vi "Servo Tracking State Machine.vi"(0 "Servo Positions In":cluster{"X":dbl, "Y":dbl}, 1 "Image Size":T4=enum."320x240", 7 "Rectangle":T3, 9 "Particles":i32, 11 "Area":i32=4) -> (4 "Servo Positions":cluster{"X":dbl, "Y":dbl}, 6 "Tracking State Info":T2)   [LabVIEW 2013]
uses:
  <vilib>/Rock Robotics/WPI/Camera/WPI_CameraImageSize.ctl
  Control States.ctl
panel:
  in  "Upper Limit":cluster{"X":i32, "Y":i32}={"X"=169, "Y"=130}
  in  "Lower Limit":cluster{"X":i32, "Y":i32}={"X"=0, "Y"=40}
  in  "Search Speed":i32=4
  in  "Proportional (div)":cluster{"X":i32, "Y":i32}={"X"=15, "Y"=-13}
  # "Unwired tuning params for control.\nSearch speed determines how fast the\ngimbal will move when trying to acquire\na target. Too fast and you may miss the\ntarget between frames, too slow is boring.\n\nProportional(div) is the proportional constant\nexpressed as a divisor term. Adjust this higher\nif the gimbal is oscillating, lower for quicker\nresponse.\n\nThe limits are useful for keeping the gimbal in\na working range, some stick when the get near\ntheir mechanical limits. It is also useful to limit\nthe searching to avoid looking at the ceiling, etc."
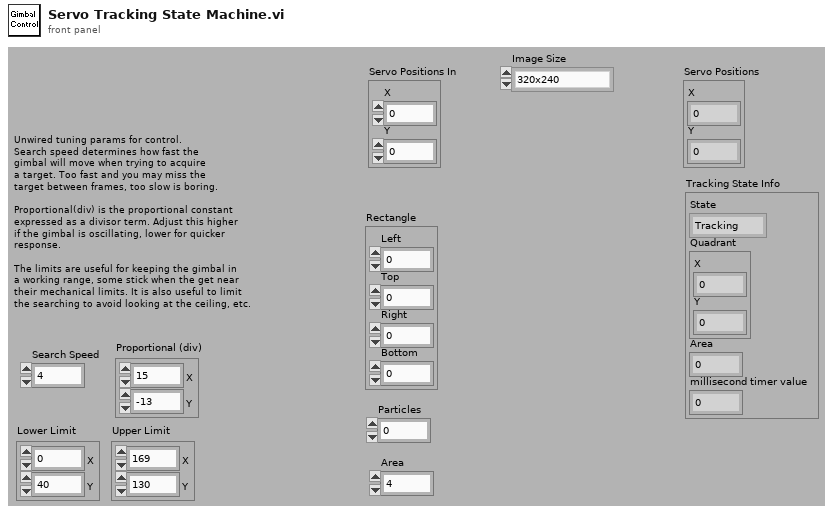
[diagram p1: front panel]
types:
  T1 = typedef "Control States.ctl" = enum16{"Tracking", "Lost Small", "Lost-Patience", "Search-Begin", "Searching", "Lost - Edge"}
  T2 = cluster{"State":T1, "Quadrant":cluster{"X":i32, "Y":i32}, "Area":i32, "millisecond timer value":u32}
  T3 = cluster{"Left":i32, "Top":i32, "Right":i32, "Bottom":i32}
  T4 = typedef "WPI_CameraImageSize.ctl" = enum16{"640x480", "320x240", "160x120"}
  T5 = cluster{"State":T1, "Grid Element":cluster{"X":i32, "Y":i32}, "Area":i32, "millisecond timer value":u32}
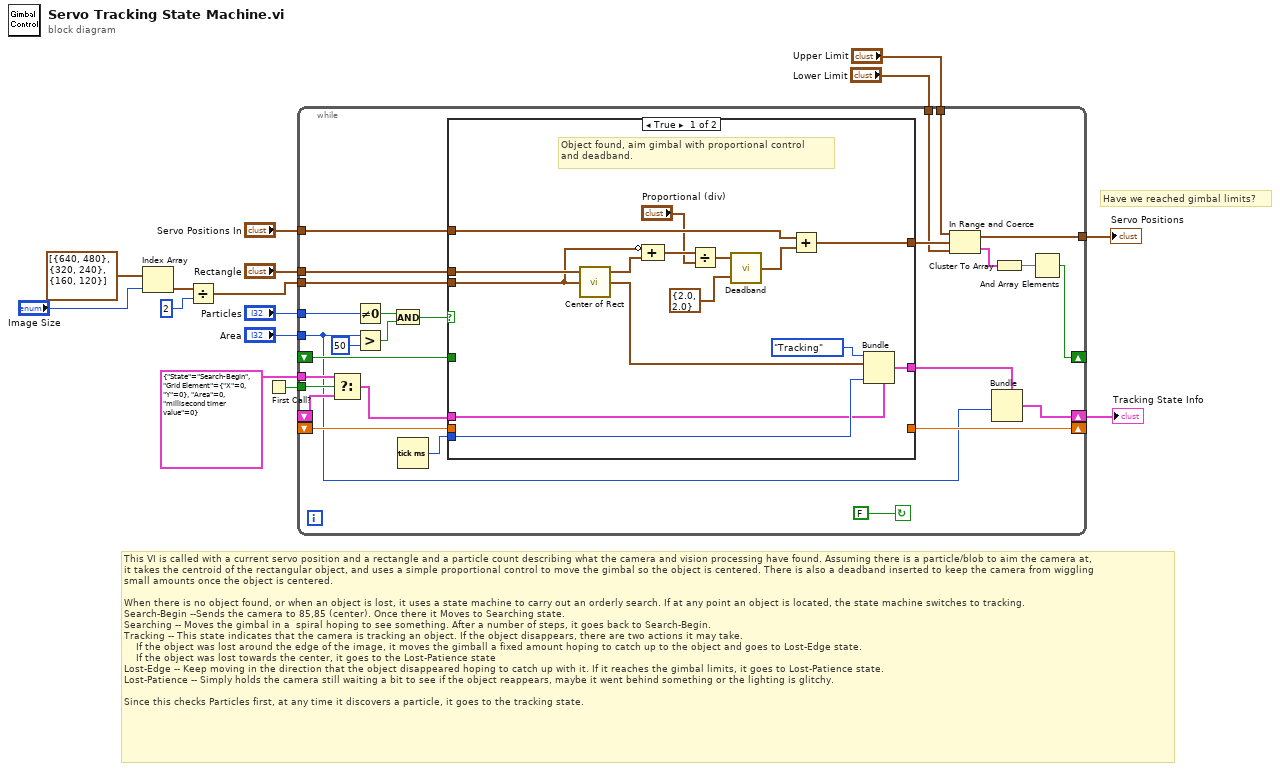
[diagram p0: block diagram]
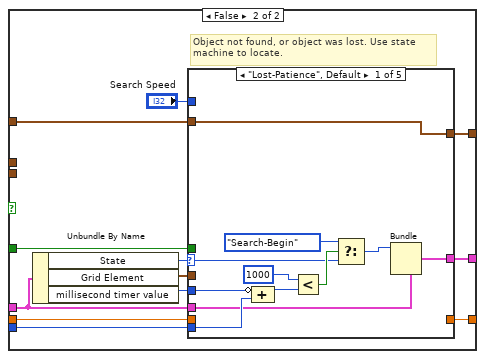
[diagram p2: hidden frame]
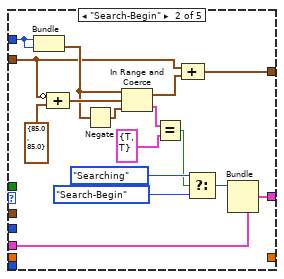
[diagram p3: hidden frame]
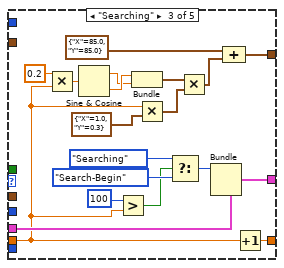
[diagram p4: hidden frame]
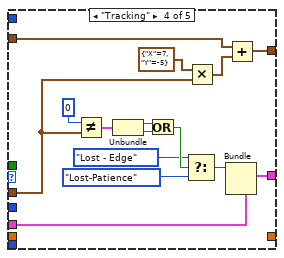
[diagram p5: hidden frame]
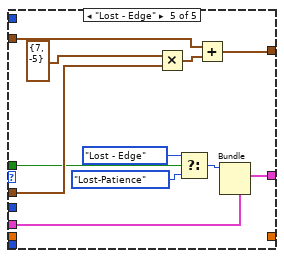
[diagram p6: hidden frame]
diagram:
  # "Have we reached gimbal limits?"
  # "This VI is called with a current servo position and a rectangle and a particle count describing what the camera and vision processing have found. Assuming there is a particle/blob to aim the camera at,\nit takes the centroid of the rectangular object, and uses a simple proportional control to move the gimbal so the object is centered. There is also a deadband inserted to keep the camera from wiggling\nsmall amounts once the object is centered.\n\nWhen there is no object found, or when an object is lost, it uses a state machine to carry out an orderly search. If at any point an object is located, the state machine switches to tracking.\nSearch-Begin --Sends the camera to 85,85 (center). Once there it Moves to Searching state.\nSearching -- Moves the gimbal in a  spiral hoping to see something. After a number of steps, it goes back to Search-Begin.\nTracking -- This state indicates that the camera is tracking an object. If the object disappears, there are two actions it may take.\n    If the object was lost around the edge of the image, it moves the gimball a fixed amount hoping to catch up to the object and goes to Lost-Edge state.\n    If the object was lost towards the center, it goes to the Lost-Patience state\nLost-Edge -- Keep moving in the direction that the object disappeared hoping to catch up with it. If it reaches the gimbal limits, it goes to Lost-Patience state.\nLost-Patience -- Simply holds the camera still waiting a bit to see if the object reappears, maybe it went behind something or the lighting is glitchy.\n\nSince this checks Particles first, at any time it discovers a particle, it goes to the tracking state."
  n1 = Index Array(array=cluster{"X":i32, "Y":i32}[] [{"X"=640, "Y"=480}, {"X"=320, "Y"=240}, {"X"=160, "Y"=120}] ("Resolutions"), index="Image Size") -> (element=w12:cluster{"X":i32, "Y":i32})
  n2 = Divide(x=w12, y=2) -> (x/y=w13:cluster{"X":dbl, "Y":dbl})
  n3 = First Call?() -> (First Call?: T/F=w5:bool)
  n4 = while {
    tunnel: w13 -> [w24]
    tunnel: "Particles" -> [w23]
    tunnel: "Rectangle" -> [w25]
    tunnel: [w33] -> w8
    shift-right: [w41] -> _
    shift-left: _ -> [w40]
    tunnel: "Servo Positions In" -> [w39]
    shift-right: [w18] -> w6
    shift-left: _ -> [w36]
    tunnel: w5 -> [w38]
    tunnel: T5 {"State"=enum."Search-Begin", "Grid Element"={"X"=0, "Y"=0}, "Area"=0, "millisecond timer value"=0} -> [w37]
    tunnel: "Lower Limit" -> [w31]
    tunnel: "Upper Limit" -> [w30]
    shift-right: [w27] -> _
    shift-left: _ -> [w26]
    tunnel: "Area" -> [w16]
    stop <- FALSE continue-if-true
    n5 = Select(t=w37, s=w38, f=w36) -> (s? t:f=w35:T5)
    n6 = Not Equal To 0?(x=w23) -> (x != 0?=w21:bool)
    n7 = Greater?(x=w16, y=50) -> (0:w20:bool)
    n8 = And(x=w21, y=w20) -> (x .and. y?=w19:bool)
    n9 = Tick Count (ms)() -> (millisecond timer value=w42:u32)
    n10 = case shown="True" w19 {
      tunnel: w25 -> [w46 _]
      tunnel: w24 -> [w43 _]
      tunnel: w42 -> [w53 w68]
      tunnel: [w55 w69] -> w17
      tunnel: w35 -> [w47 w61]
      tunnel: w39 -> [w54 w66]
      tunnel: [w52 w67] -> w32
      tunnel: w40 -> [_ w65]
      tunnel: [_ w64] -> w41
      tunnel: w26 -> [_ w63]
      frame True {
        # "Object found, aim gimbal with proportional control\nand deadband."
        n11 = call "Center of Rect.vi"("Camera Center"=w43, "Rectangle"=w46) -> ("Grid Element"=w44:cluster{"X":i32, "Y":i32}, "Center"=w45:cluster{dbl, dbl})  [unwired: 1 in, 1 out]
        n12 = Compound Arithmetic op=ADD(invert w43, w45) -> (w57:cluster{dbl, dbl})
        n13 = Divide(x=w57, y="Proportional (div)") -> (x/y=w50:cluster{dbl, dbl})
        n14 = call "Deadband.vi"("Deadband"=cluster{dbl, dbl} {2.0, 2.0}, "Value"=w50) -> ("Value Out"=w49:cluster{dbl, dbl})
        n15 = Add(x=w54, y=w49) -> (x+y=w52:cluster{dbl, dbl})
        n16 = Bundle(cluster=w47, "State"=Control_States."Tracking", "Grid Element"=w44, "millisecond timer value"=w53) -> (w55:T5)  [unwired: 1 out]
      }
      frame False {
        # "Object not found, or object was lost. Use state\nmachine to locate."
        n17 = Unbundle By Name(w61) -> ("State"=w60:T1, "Grid Element"=w59:cluster{"X":i32, "Y":i32}, "millisecond timer value"=w58:u32)
        n18 = case shown="\"Lost-Patience\", Default" w60 {
          selector: w60 -> [w71 _ _ _ _]
          tunnel: [w72 w87 w102 w130 w141] -> w69
          tunnel: w61 -> [w76 w88 w103 w129 w140]
          tunnel: w58 -> [w79 _ _ _ _]
          tunnel: w68 -> [w80 _ _ _ _]
          tunnel: [w70 w89 w107 w121 w136] -> w67
          tunnel: w66 -> [w70 w90 _ w120 w137]
          tunnel: "Search Speed" -> [_ w94 _ _ _]
          tunnel: w65 -> [_ _ w98 _ _]
          tunnel: [_ _ w115 _ _] -> w64
          tunnel: w59 -> [_ _ _ w117 w135]
          tunnel: w63 -> [_ _ _ _ w131]
          frame "Lost-Patience", Default {
            n19 = Compound Arithmetic op=ADD(invert w79, w80) -> (w78:u32)
            n20 = Less?(x=1000, y=w78) -> (x < y?=w73:bool)
            n21 = Select(t=Control_States."Search-Begin" ("State"), s=w73, f=w71) -> (s? t:f=w75:T1)
            n22 = Bundle(cluster=w76, "State"=w75) -> (w72:T5)  [unwired: 3 out]
          }
          frame "Search-Begin" {
            n23 = Bundle("Search Speed"=w94, "Search Speed"=w94) -> (w93:cluster{"Search Speed":i32, "Search Speed":i32})  [unwired: 1 out]
            n24 = Compound Arithmetic op=ADD(invert w90, cluster{"X":dbl, "Y":dbl} {"X"=85.0, "Y"=85.0} ("Servos")) -> (w95:cluster{"X":dbl, "Y":dbl})
            n25 = Negate(x=w93) -> (-x=w92:cluster{"Search Speed":i32, "Search Speed":i32})
            n26 = In Range and Coerce(upper limit=w93, x=w95, lower limit=w92) -> (coerced(x)=w91:cluster{"X":dbl, "Y":dbl}, In Range?=w83:cluster{"X":bool, "Y":bool})
            n27 = Equal?(x=w83, y=cluster{"X":bool, "Y":bool} {"X"=TRUE, "Y"=TRUE}) -> (x = y?=w81:bool)
            n28 = Compound Arithmetic op=ADD(w90, w91) -> (w89:cluster{"X":dbl, "Y":dbl})
            n29 = Select(t=Control_States."Searching" ("State"), s=w81, f=Control_States."Search-Begin" ("State")) -> (s? t:f=w86:T1)
            n30 = Bundle(cluster=w88, "State"=w86) -> (w87:T5)  [unwired: 3 out]
          }
          frame "Searching" {
            n31 = Multiply(x=0.2, y=w98) -> (x*y=w113:dbl)
            n32 = Sine & Cosine(0:w113) -> (1:w111:dbl, 2:w112:dbl)
            n33 = Greater?(x=100, y=w98) -> (0:w100:bool)
            n34 = Bundle(w112, w111) -> (w110:cluster{dbl, dbl})  [unwired: 1 out]
            n35 = Multiply(x=w98, y=cluster{"X":dbl, "Y":dbl} {"X"=1.0, "Y"=0.3} ("Servos")) -> (x*y=w99:cluster{"X":dbl, "Y":dbl})
            n36 = Select(t=Control_States."Searching" ("State"), s=w100, f=Control_States."Search-Begin" ("State")) -> (s? t:f=w106:T1)
            n37 = Multiply(x=w110, y=w99) -> (x*y=w109:cluster{dbl, dbl})
            n38 = Bundle(cluster=w103, "State"=w106) -> (w102:T5)  [unwired: 3 out]
            n39 = Compound Arithmetic op=ADD(cluster{"X":dbl, "Y":dbl} {"X"=85.0, "Y"=85.0} ("Servos"), w109) -> (w107:cluster{dbl, dbl})
            n40 = Increment(x=w98) -> (x+1=w115:dbl)
          }
          frame "Tracking" {
            n41 = Not Equal?(x=0 ("X"), y=w117) -> (x != y?=w128:cluster{"X":bool, "Y":bool})
            n42 = Unbundle(w128) -> ("X"=w127:bool, "Y"=w126:bool)
            n43 = Or(x=w127, y=w126) -> (x .or. y?=w125:bool)
            n44 = Select(t=Control_States."Lost - Edge" ("State"), s=w125, f=Control_States."Lost-Patience" ("State")) -> (s? t:f=w122:T1)
            n45 = Multiply(x=cluster{"X":i32, "Y":i32} {"X"=7, "Y"=-5}, y=w117) -> (x*y=w119:cluster{"X":i32, "Y":i32})
            n46 = Bundle(cluster=w129, "State"=w122) -> (w130:T5)  [unwired: 3 out]
            n47 = Add(x=w120, y=w119) -> (x+y=w121:cluster{"X":dbl, "Y":dbl})
          }
          frame "Lost - Edge" {
            n48 = Multiply(x=cluster{"X":i32, "Y":i32} {"X"=7, "Y"=-5}, y=w135) -> (x*y=w139:cluster{"X":i32, "Y":i32})
            n49 = Select(t=Control_States."Lost - Edge" ("State"), s=w131, f=Control_States."Lost-Patience" ("State")) -> (s? t:f=w134:T1)
            n50 = Add(x=w137, y=w139) -> (x+y=w136:cluster{"X":dbl, "Y":dbl})
            n51 = Bundle(cluster=w140, "State"=w134) -> (w141:T5)  [unwired: 3 out]
          }
        }
      }
    }
    n52 = In Range and Coerce(upper limit=w30, x=w32, lower limit=w31) -> (coerced(x)=w33:cluster{"X":dbl, "Y":dbl}, In Range?=w29:cluster{"X":bool, "Y":bool})
    n53 = Bundle(cluster=w17, "Area"=w16) -> (w18:T5)  [unwired: 3 out]
    n54 = Cluster To Array(cluster=w29) -> (array=w28:bool[])
    n55 = And Array Elements(Boolean array=w28) -> (logical AND=w27:bool)
  }
  "Servo Positions" <- w8
  "Tracking State Info" <- w6
